vi "Write Done.vi"(8 "error in (no error)":errorcluster, 9 "Bytes":u64, 10 "Time":dbl, 11 "Main in":refnum<class "Main.lvclass">) -> (0 "error out":errorcluster, 3 "Main out":refnum<class "Main.lvclass">)   [LabVIEW 2025, in "Main.lvlib" / "Main.lvclass"]
uses:
  Main.lvclass
  Main.lvclass/Main.ctl
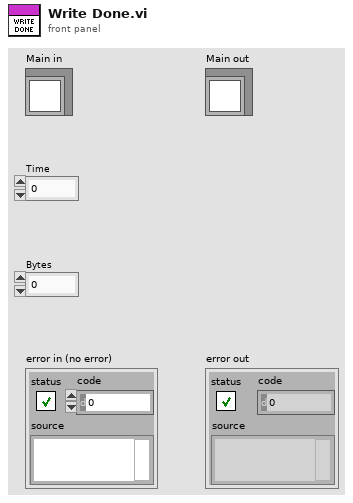
[diagram p1: front panel]
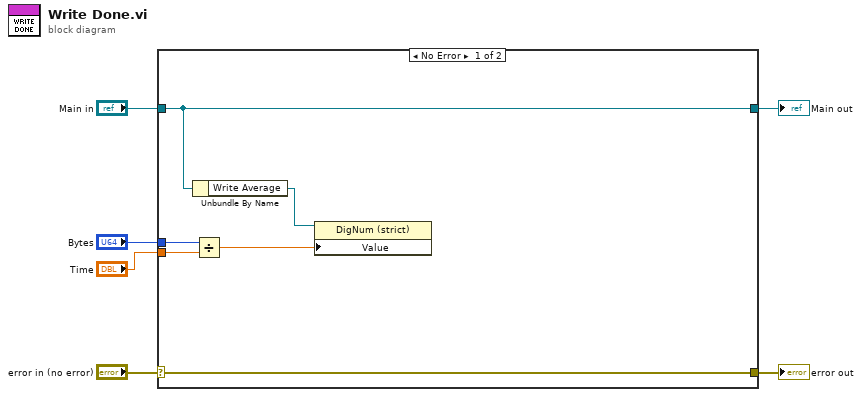
[diagram p0: block diagram]
diagram:
  n1 = case shown="No Error" "error in (no error)" {
    selector: "error in (no error)" -> [w12 w14]
    tunnel: [w12 w14] -> w5
    tunnel: [w8 w13] -> w3
    tunnel: "Main in" -> [w8 w13]
    tunnel: "Bytes" -> [w11 _]
    tunnel: "Time" -> [w10 _]
    frame No Error {
      n2 = Unbundle By Name(w8) -> ("Write Average"=w7:refnum<vi>)
      n3 = Divide(x=w11, y=w10) -> (x/y=w9:dbl)
      n4 = property class="DigNum (strict)"(reference=w7, "Value"=w9) -> ()  [unwired: 1 in, 2 out]
    }
    frame Error {
    }
  }
  "error out" <- w5
  "Main out" <- w3
